vi "Copy One page.vi"(0 "PDFCopy IN":refnum<k24>, 5 "PDF Document IN":refnum<k24>, 7 "PdfReader IN":refnum<k24>, 9 "index":i32, 11 "error in (no error)":errorcluster) -> (4 "PDFCopy OUT":refnum<k24>, 6 "PDF Document OUT":refnum<k24>, 8 "PdfReader OUT":refnum<k24>, 10 "GetPageSizeWithRotation":refnum<k24>, 15 "error out":errorcluster)   [LabVIEW 2019, in "Exaprom PDF.lvlib"]
doc: "Version 1.1\nDeveloped by Jean-Marc Simard\nCopyright © 2012, Exaprom Inc.\nAll rights reserved.\nLicense: BSD\n\nWith iTextSharp 4.1.6 (http://itextsharp.sourceforge.net)\nunder Mozilla Public License Version 1.1\n(http://www.mozilla.org/MPL/MPL-1.1.html)"
uses:
  C:/work/niobrara_lv/labview pdf writer fixing/DLL/itextsharp.dll
  DLL/itextsharp.dll
  Exaprom PDF.lvlib
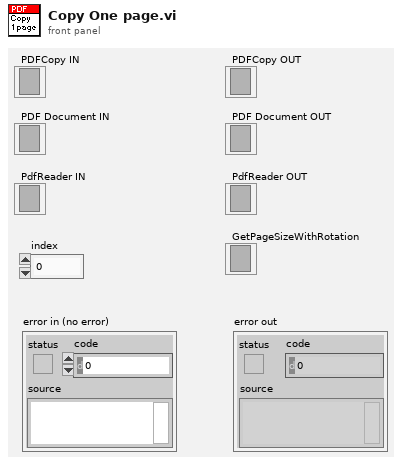
[diagram p1: front panel]
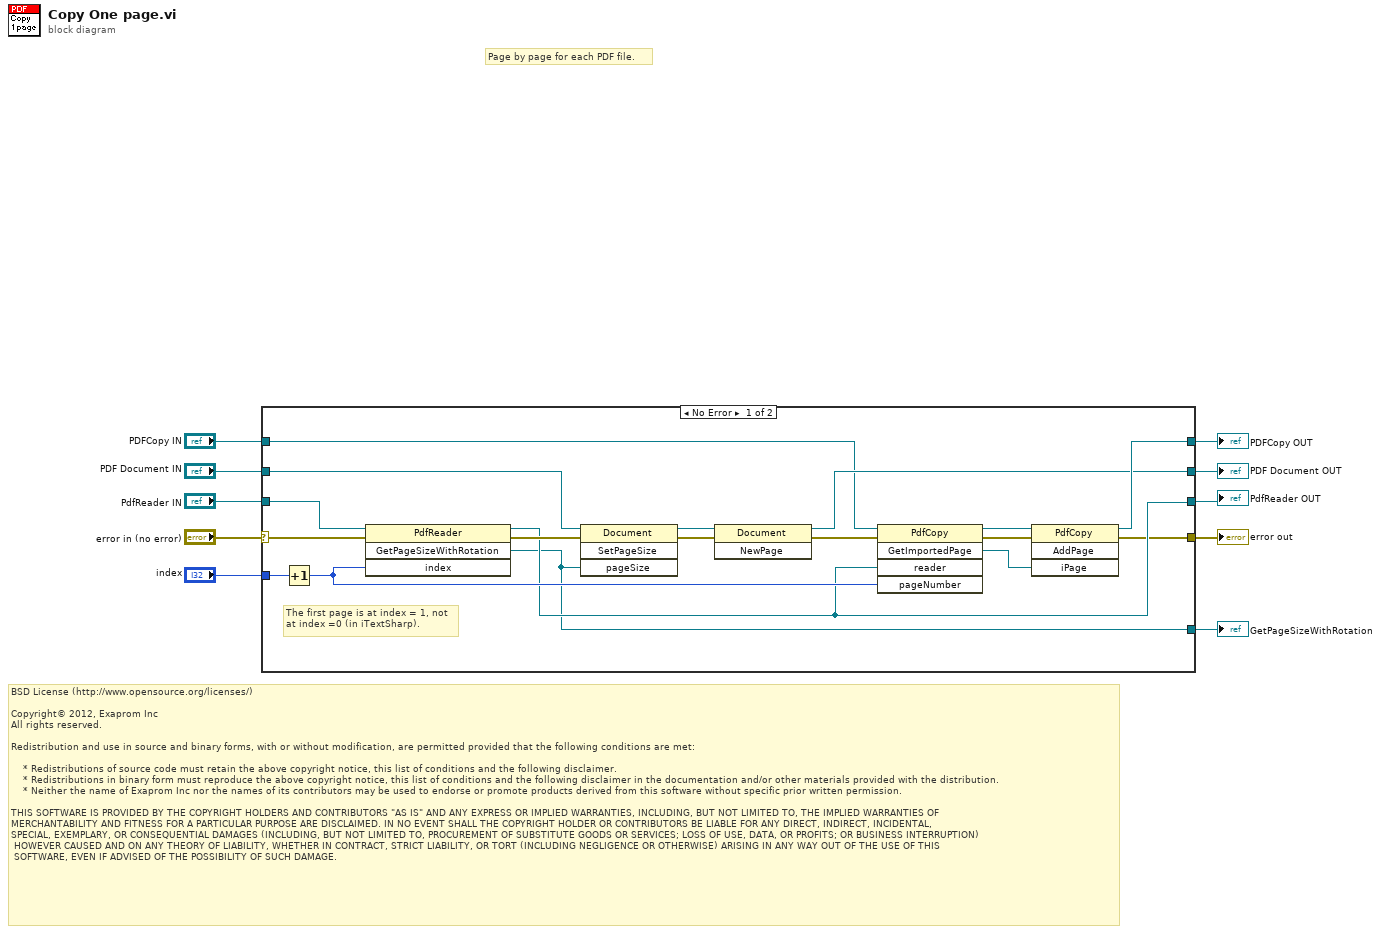
[diagram p0: block diagram]
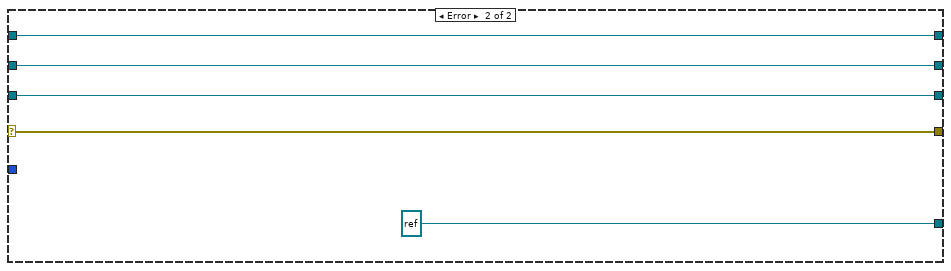
[diagram p2: hidden frame]
diagram:
  # "Page by page for each PDF file."
  # "BSD License (http://www.opensource.org/licenses/)\n\nCopyright© 2012, Exaprom Inc\nAll rights reserved.\n\nRedistribution and use in source and binary forms, with or without modification, are permitted provided that the following conditions are met:\n\n    * Redistributions of source code must retain the above copyright notice, this list of conditions and the following disclaimer.\n    * Redistributions in binary form must reproduce the above copyright notice, this list of conditions and the following disclaimer in the documentation and/or other materials provided with the distribution.\n    * Neither the name of Exaprom Inc nor the names of its contributors may be used to endorse or promote products derived from this software without specific prior written permission.\n\nTHIS SOFTWARE IS PROVIDED BY THE COPYRIGHT HOLDERS AND CONTRIBUTORS \"AS IS\" AND ANY EXPRESS OR IMPLIED WARRANTIES, INCLUDING, BUT NOT LIMITED TO, THE IMPLIED WARRANTIES OF \nMERCHANTABILITY AND FITNESS FOR A PARTICULAR PURPOSE ARE DISCLAIMED. IN NO EVENT SHALL THE COPYRIGHT HOLDER OR CONTRIBUTORS BE LIABLE FOR ANY DIRECT, INDIRECT, INCIDENTAL,\nSPECIAL, EXEMPLARY, OR CONSEQUENTIAL DAMAGES (INCLUDING, BUT NOT LIMITED TO, PROCUREMENT OF SUBSTITUTE GOODS OR SERVICES; LOSS OF USE, DATA, OR PROFITS; OR BUSINESS INTERRUPTION)\n HOWEVER CAUSED AND ON ANY THEORY OF LIABILITY, WHETHER IN CONTRACT, STRICT LIABILITY, OR TORT (INCLUDING NEGLIGENCE OR OTHERWISE) ARISING IN ANY WAY OUT OF THE USE OF THIS\n SOFTWARE, EVEN IF ADVISED OF THE POSSIBILITY OF SUCH DAMAGE."
  n1 = case shown="No Error" "error in (no error)" {
    selector: "error in (no error)" -> [w23 w33]
    tunnel: [w17 w33] -> w10
    tunnel: [w22 w32] -> w8
    tunnel: "PdfReader IN" -> [w21 w32]
    tunnel: "index" -> [w20 _]
    tunnel: "PDF Document IN" -> [w19 w31]
    tunnel: [w12 w31] -> w4
    tunnel: "PDFCopy IN" -> [w11 w30]
    tunnel: [w18 w30] -> w2
    tunnel: [w14 refnum<k24> refnum ("GetPageSizeWithRotation")] -> w1
    frame No Error {
      # "The first page is at index = 1, not\nat index =0 (in iTextSharp)."
      n2 = Increment(x=w20) -> (x+1=w25:i32)
      n3 = invoke class="PdfReader" method="GetPageSizeWithRotation"(reference=w21, error in=w23, "index"=w25) -> (reference out=w22:refnum<k24>, error out=w24:errorcluster, "GetPageSizeWithRotation"=w14:refnum<k24>)  [unwired: 1 in, 1 out]
      n4 = invoke class="Document" method="SetPageSize"(reference=w19, error in=w24, "pageSize"=w14) -> (reference out=w13:refnum<k24>, error out=w15:errorcluster)  [unwired: 1 in, 2 out]
      n5 = invoke class="Document" method="NewPage"(reference=w13, error in=w15) -> (reference out=w12:refnum<k24>, error out=w16:errorcluster)  [unwired: 1 in, 1 out]
      n6 = invoke class="PdfCopy" method="GetImportedPage"(reference=w11, error in=w16, "reader"=w22, "pageNumber"=w25) -> (reference out=w28:refnum<k24>, error out=w26:errorcluster, "GetImportedPage"=w27:refnum<k24>)  [unwired: 1 in, 2 out]
      n7 = invoke class="PdfCopy" method="AddPage"(reference=w28, error in=w26, "iPage"=w27) -> (reference out=w18:refnum<k24>, error out=w17:errorcluster)  [unwired: 1 in, 2 out]
    }
    frame Error {
    }
  }
  "error out" <- w10
  "PdfReader OUT" <- w8
  "PDF Document OUT" <- w4
  "PDFCopy OUT" <- w2
  "GetPageSizeWithRotation" <- w1
